vi "Scripting_WireTerminals.vi"(8 "error in":errorcluster, 9 "CleanUpWire(True)":bool=TRUE, 10 "Term 2":refnum<vi>, 11 "Term 1":refnum<vi>) -> (0 "error out":errorcluster)   [LabVIEW 2020]
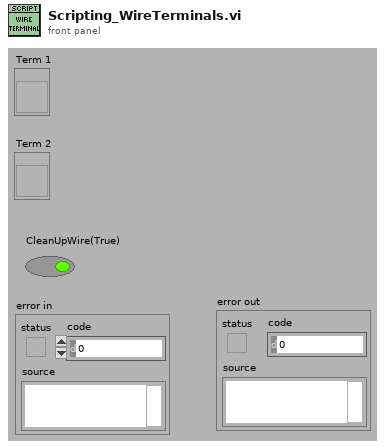
[diagram p1: front panel]
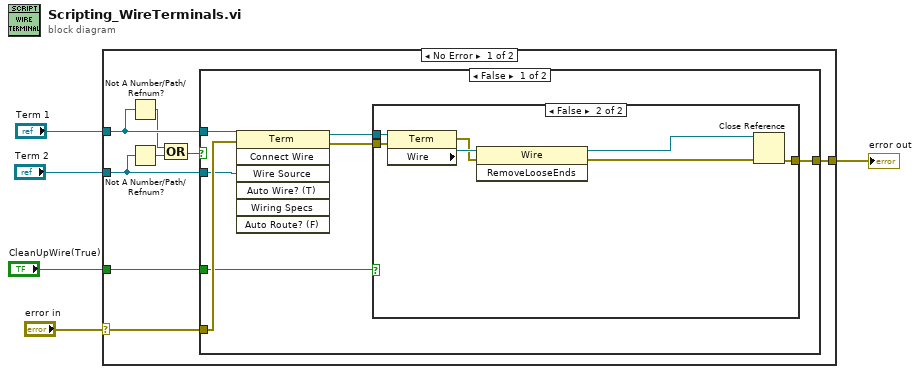
[diagram p0: block diagram]
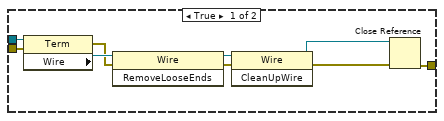
[diagram p2: hidden frame]
diagram:
  n1 = case shown="No Error" "error in" {
    selector: "error in" -> [w12 w38]
    tunnel: "Term 2" -> [w9 _]
    tunnel: "Term 1" -> [w10 _]
    tunnel: [w13 w38] -> w3
    tunnel: "CleanUpWire(True)" -> [w11 _]
    frame No Error {
      n2 = Not A Number/Path/Refnum?(number/path/refnum=w10) -> (NaN/Path/Refnum?=w7:bool)
      n3 = Not A Number/Path/Refnum?(number/path/refnum=w9) -> (NaN/Path/Refnum?=w8:bool)
      n4 = Compound Arithmetic op=OR(w7, w8) -> (w6:bool)
      n5 = case shown="False" w6 {
        tunnel: [w18 w37] -> w13
        tunnel: w12 -> [w17 w37]
        tunnel: w11 -> [w16 _]
        tunnel: w10 -> [w15 _]
        tunnel: w9 -> [w14 _]
        frame False {
          n6 = invoke class="Term" method="Connect Wire"(reference=w15, error in=w17, "Wire Source"=w14) -> (reference out=w20:refnum<vi>, error out=w19:errorcluster)  [unwired: 4 in, 5 out]
          n7 = case shown="False" w16 {
            tunnel: w20 -> [w29 w36]
            tunnel: w19 -> [w28 w35]
            tunnel: [w25 w34] -> w18
            frame True {
              n8 = property class="Term"(reference=w29, error in=w28) -> (error out=w23:errorcluster, "Wire"=w24:refnum<vi>)  [unwired: 1 out]
              n9 = invoke class="Wire" method="RemoveLooseEnds"(reference=w24, error in=w23) -> (reference out=w22:refnum<vi>, error out=w21:errorcluster)  [unwired: 1 in, 1 out]
              n10 = invoke class="Wire" method="CleanUpWire"(reference=w22, error in=w21) -> (reference out=w26:refnum<vi>, error out=w27:errorcluster)  [unwired: 1 in, 1 out]
              n11 = Close Reference(reference=w26, error in (no error)=w27) -> (error out=w25:errorcluster)
            }
            frame False {
              n12 = property class="Term"(reference=w36, error in=w35) -> (error out=w32:errorcluster, "Wire"=w33:refnum<vi>)  [unwired: 1 out]
              n13 = invoke class="Wire" method="RemoveLooseEnds"(reference=w33, error in=w32) -> (reference out=w30:refnum<vi>, error out=w31:errorcluster)  [unwired: 1 in, 1 out]
              n14 = Close Reference(reference=w30, error in (no error)=w31) -> (error out=w34:errorcluster)
            }
          }
        }
        frame True {
        }
      }
    }
    frame Error {
    }
  }
  "error out" <- w3
